vi "System Mapping Tool Main.vi"() -> ()   [LabVIEW 2016, in "System Mapping Tool.lvlib"]
uses:
  NationalInstruments.VeriStand.SystemStorageUI
  System Mapping Tool.lvlib
panel:
  in  "Load SDF 6":bool
  in  "Load SDF 5":bool
  in  "Load SDF 4":bool
  in  "Load SDF 3":bool
  in  "Load SDF 2":bool
  in  "Load SDF":bool
  in  "Sources":refnum<k24>(container)
  in  "Load SDF 7":bool
  in  "Destinations":refnum<k24>(container)
  in  "Mappings":T1(tab)
  in  "Mappings":i32(listbox)
  in  "Filter":string
  in  "Filter Mode":enum32{"By Source", "By Destination"}(radio)
  in  "Mappings 2":i32(listbox)
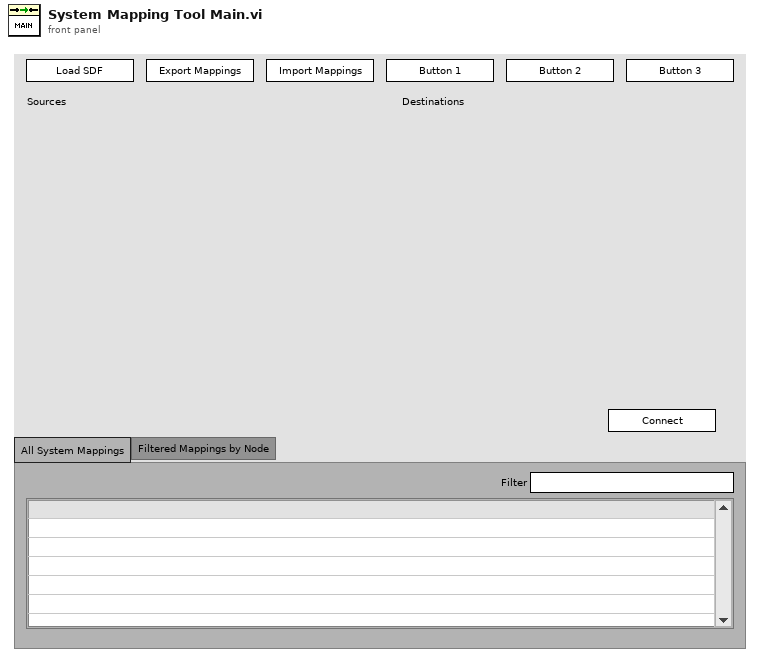
[diagram p1: front panel]
types:
  T1 = enum32{"All System Mappings", "Filtered Mappings by Node"}
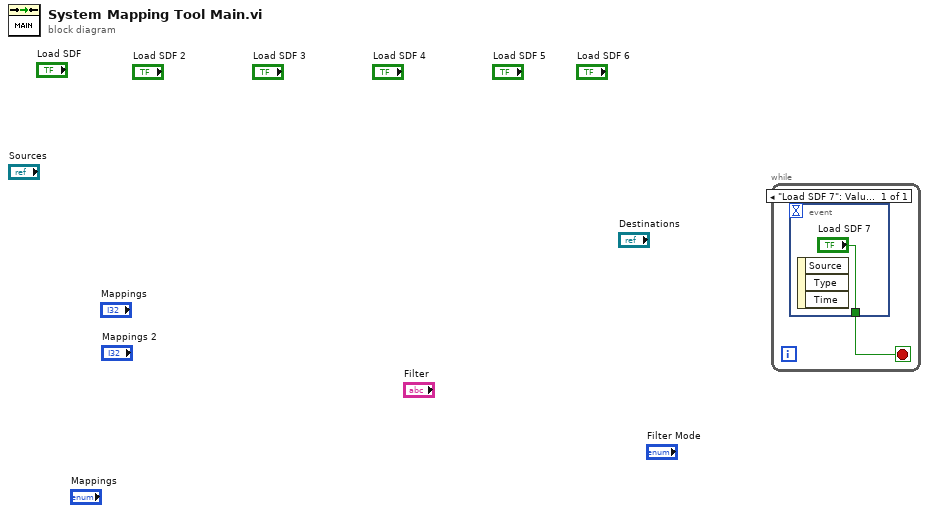
[diagram p0: block diagram]
diagram:
  n1 = while {
    stop <- w1 stop-if-true
    n2 = event shown="[0] \"Load SDF 7\": Value Change" {
      selector: _ -> [_]
      dyn-events: _ -> [_]
      timeout: _ -> [_]
      tunnel: ["Load SDF 7"] -> w1
      event "Load SDF 7": Value Change {
        n3 = event-data() -> ()  [unwired: 1 in, 3 out]
      }
    }
  }
